vi "Get Test Data.vi"(8 "error in":errorcluster, 10 "Data":T1, 11 "CRDS in":refnum<class "CRDS.lvclass">) -> (0 "error out":errorcluster, 3 "CRDS out":refnum<class "CRDS.lvclass">)   [LabVIEW 2015, in "CRDS.lvclass"]
uses:
  Main/CRDS.lvclass
  Data/Cell/calData.ctl
  Main/CRDS.lvclass/CRDS.ctl
  Data/Write measTime.vi
  Data/Main/Read CellData.vi
  Data/Main/Write filter.vi
  Data/Cell/Write hkParam.vi
  Data/Main/Write CellData.vi
  Data/Cell/CRDS Cell Data.lvclass
  Data/Main/CRDS Data.lvclass
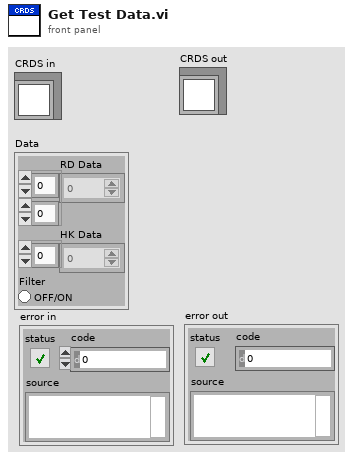
[diagram p1: front panel]
types:
  T1 = cluster{"RD Data":dbl[][], "HK Data":dbl[], "Filter":bool}
  T2 = typedef "calData.ctl" = cluster{"rhDilFac":sgl, "Q":sgl, "Tmean":sgl, "extDilFac":sgl, "rhCell":sgl, "P":sgl, "T":sgl}
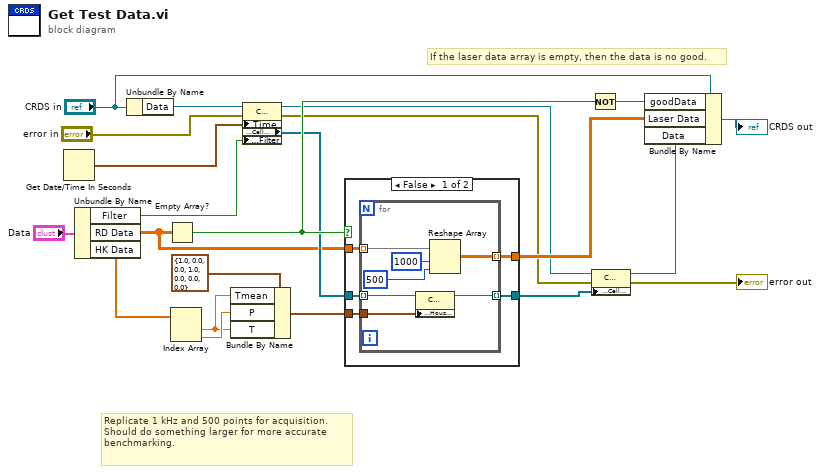
[diagram p0: block diagram]
diagram:
  # "If the laser data array is empty, then the data is no good."
  # "Replicate 1 kHz and 500 points for acquisition.  Should do something larger for more accurate benchmarking."
  n1 = Get Date/Time In Seconds() -> (seconds since 1Jan1904=w9:timestamp)
  n2 = Unbundle By Name("Data") -> ("Filter"=w13:bool, "RD Data"=w3:dbl[][], "HK Data"=w2:dbl[])
  n3 = Unbundle By Name("CRDS in") -> ("Data"=w8:refnum<class "CRDS Data.lvclass">)
  n4 = Empty Array?(array=w3) -> (empty?=w20:bool)
  n5 = Index Array(array=w2) -> (element #1=w16:dbl, element #2=w17:dbl)  [unwired: 2 in]
  n6 = Bundle By Name(cluster=T2 {"rhDilFac"=1.0, "Q"=0.0, "Tmean"=0.0, "extDilFac"=1.0, "rhCell"=0.0, "P"=0.0, "T"=0.0} ("Housekeeping"), "Tmean"=w16, "P"=w17, "T"=w16) -> (w18:T2)
  n7 = property class="CRDS"(reference=w8, error in="error in", "Time"=w9, "Data Access:Filter"=w13) -> (reference out=w10:refnum<class "CRDS Data.lvclass">, error out=w5:errorcluster, "Data Access:Cell Data"=w14:refnum<class "CRDS Cell Data.lvclass">[])
  n8 = case shown="False" w20 {
    tunnel: w14 -> [w27 w35]
    tunnel: w18 -> [w26 _]
    tunnel: [w25 w35] -> w19
    tunnel: w3 -> [w24 _]
    tunnel: [w23 _] -> w22
    frame False {
      n9 = for {
        tunnel: w27 -> [w34] mode=indexing
        tunnel: w24 -> [w33] mode=indexing
        tunnel: [w30] -> w25 mode=indexing
        tunnel: w26 -> [w29]
        tunnel: [w28] -> w23 mode=indexing
        n10 = property class="CRDS Cell"(reference=w34, "Data Access:Housekeeping"=w29) -> (reference out=w30:refnum<class "CRDS Cell Data.lvclass">)  [unwired: 1 in, 1 out]
        n11 = Reshape Array(w33, 1000 ("dimension size"), 500 ("dimension size")) -> (w28:dbl[][])
      }
    }
    frame True {
    }
  }
  n12 = Not(x=w20) -> (.not. x?=w21:bool)
  n13 = property class="CRDS"(reference=w10, error in=w5, "Data Access:Cell Data"=w19) -> (reference out=w1:refnum<class "CRDS Data.lvclass">, error out=→"error out":errorcluster)
  n14 = Bundle By Name(cluster="CRDS in", "goodData"=w21, "Laser Data"=w22, "Data"=w1) -> (→"CRDS out":refnum<class "CRDS.lvclass">)
